vi "100.vi"() -> ()   [LabVIEW 2019]
panel:
  out "난수 101":dbl
  out "Waveform Chart 2":dbl(graph)
  out "Waveform Chart":dbl(graph)
  out "난수 100":dbl
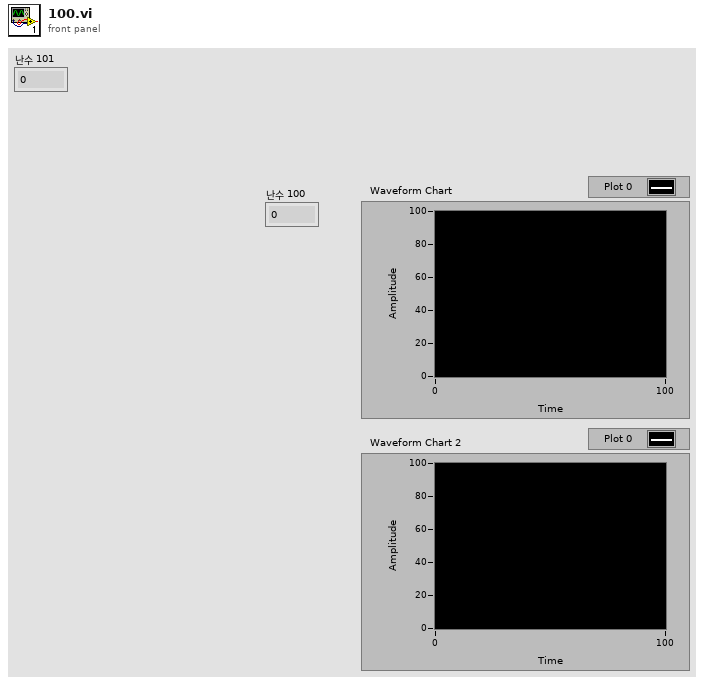
[diagram p1: front panel]
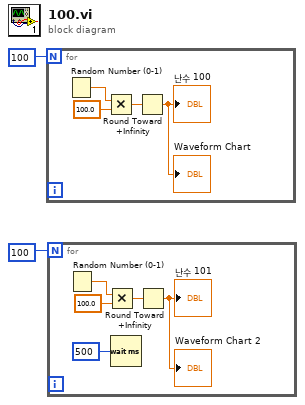
[diagram p0: block diagram]
diagram:
  n1 = for {
    N: 100 -> [_]
    n2 = Random Number (0-1)() -> (number: 0 to 1=w6:dbl)
    n3 = Multiply(x=w6, y=100.0) -> (x*y=w5:dbl)
    n4 = Round Toward +Infinity(x=w5) -> (ceil(x): smallest int >= x=→"난수 100" →"Waveform Chart":dbl)
  }
  n5 = for {
    N: 100 -> [_]
    n6 = Random Number (0-1)() -> (number: 0 to 1=w11:dbl)
    n7 = Multiply(x=w11, y=100.0) -> (x*y=w10:dbl)
    n8 = Wait (ms)(milliseconds to wait=500) -> ()  [unwired: 1 out]
    n9 = Round Toward +Infinity(x=w10) -> (ceil(x): smallest int >= x=→"난수 101" →"Waveform Chart 2":dbl)
  }
